vi "countOccurrence.vi"(8 "errorIn":errorcluster, 10 "keyword":string="Specjalista (Mid / Regular)", 11 "dataArray":string[](array[string])) -> (0 "errorOut":errorcluster, 3 "amount":dbl)   [LabVIEW 2025]
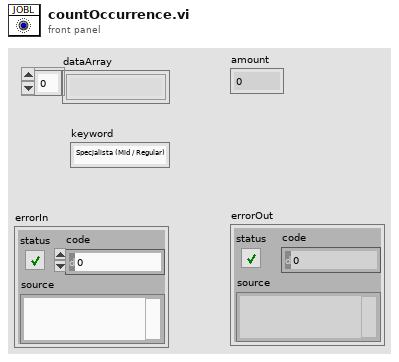
[diagram p1: front panel]
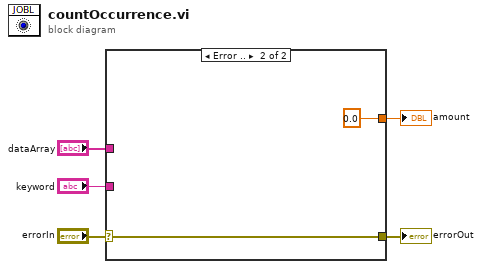
[diagram p0: block diagram]
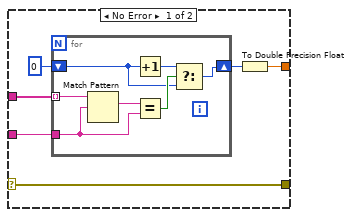
[diagram p2: hidden frame]
diagram:
  n1 = case shown="Error .." "errorIn" {
    selector: "errorIn" -> [w10 w20]
    tunnel: [w10 w20] -> w4
    tunnel: [w6 0.0] -> w3
    tunnel: "keyword" -> [w9 _]
    tunnel: "dataArray" -> [w8 _]
    frame No Error {
      n2 = for {
        tunnel: w8 -> [w18] mode=indexing
        shift-right: [w13] -> w7
        shift-left: 0 -> [w14]
        tunnel: w9 -> [w12]
        n3 = Match Pattern(string=w18, regular expression=w12) -> (match substring=w17:string)  [unwired: 1 in, 3 out]
        n4 = Increment(x=w14) -> (x+1=w15:i32)
        n5 = Equal?(x=w17, y=w12) -> (x = y?=w16:bool)
        n6 = Select(t=w15, s=w16, f=w14) -> (s? t:f=w13:i32)
      }
      n7 = To Double Precision Float(number=w7) -> (double precision float=w6:dbl)
    }
    frame Error {
    }
  }
  "errorOut" <- w4
  "amount" <- w3
